vi "FullAlign.vi"(0 "Joystick 0":dbl, 1 "Button":bool=TRUE, 5 "Joystick 1":dbl, 7 "Distance":dbl=-10000.0, 9 "Angle":dbl=-292.57472985881094) -> (4 "Right Motor":dbl=-0.2, 6 "Left Motor":dbl=0.2, 10 "Not In Sight?":bool=TRUE, 15 "In Range?":bool)   [LabVIEW 2016]
uses:
  Systems/Global 1.vi
panel:
  in  "Forward Speed":dbl=0.3 format="%#_13g"
  in  "Max Error":dbl=100.0 format="%#_13g"
  in  "Turn_Gain":dbl=0.25 format="%#_13g"
  in  "Align Effort Addition":dbl=0.175 min=0.0 max=1.0 step=0.05 format="%#_13g"
  in  "Align Target":dbl format="%#_13g"
  in  "MinDistance":dbl=24.0 format="%#_13g"
  out "Sees Target?":bool
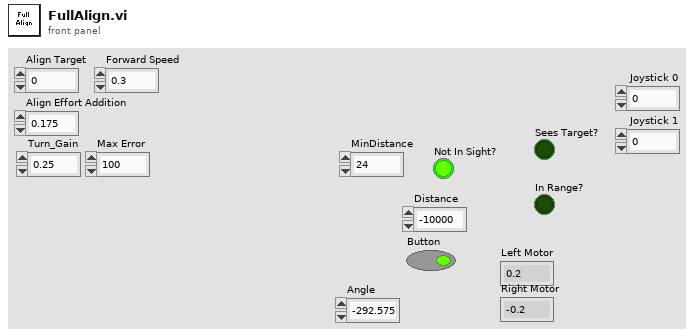
[diagram p1: front panel]
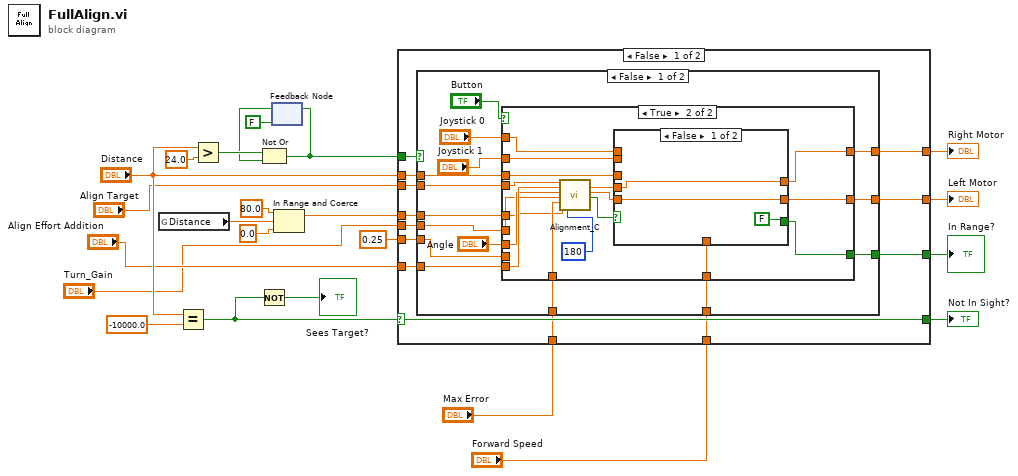
[diagram p0: block diagram]
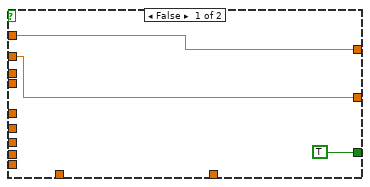
[diagram p2: hidden frame]
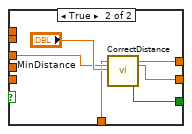
[diagram p3: hidden frame]
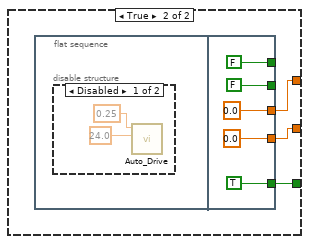
[diagram p4: hidden frame]
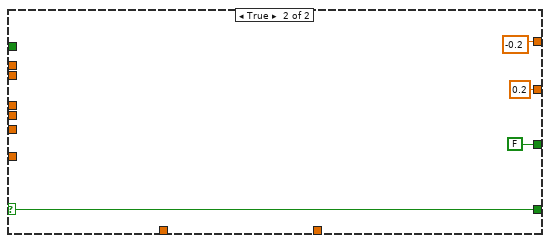
[diagram p6: hidden frame]
diagram:
  n1 = global read "Global 1.vi" "Distance"() -> (w10:dbl)
  n2 = Equal?(x="Distance", y=-10000.0) -> (x = y?=w11:bool)
  n3 = Greater?(x="Distance", y=24.0) -> (0:w16:bool)
  n4 = Not(x=w11) -> (.not. x?=→"Sees Target?":bool)
  n5 = feedback #1(FALSE) -> (w15:bool)
  n6 = Not Or(1:w15, 2:w16) -> (0:w17:bool)
  n7 = feedback-in #1(w17) -> ()
  n8 = In Range and Coerce(upper limit=80.0, x=w10, lower limit=0.0) -> (coerced(x)=w7:dbl)  [unwired: 1 out]
  n9 = case shown="False" w11 {
    selector: w11 -> [w29 w92]
    tunnel: w17 -> [w36 _]
    tunnel: [w35 -0.2] -> w22
    tunnel: [w34 0.2] -> w12
    tunnel: [w33 FALSE] -> w18
    tunnel: "Distance" -> [w32 _]
    tunnel: 0.25 -> [w31 _]
    tunnel: w7 -> [w30 _]
    tunnel: [w29 w92] -> w6
    tunnel: "Align Target" -> [w28 _]
    tunnel: "Align Effort Addition" -> [w27 _]
    tunnel: "Turn_Gain" -> [w26 _]
    tunnel: "Max Error" -> [w25 _]
    tunnel: "Forward Speed" -> [w24 _]
    frame False {
      n10 = case shown="False" w36 {
        tunnel: w32 -> [w47 _]
        tunnel: [w46 w82] -> w35
        tunnel: [w45 w81] -> w34
        tunnel: [w44 w83] -> w33
        tunnel: w31 -> [w43 _]
        tunnel: w30 -> [w42 _]
        tunnel: w28 -> [w41 _]
        tunnel: w27 -> [w40 _]
        tunnel: w26 -> [w39 _]
        tunnel: w25 -> [w38 _]
        tunnel: w24 -> [w37 _]
        frame False {
          n11 = case shown="True" "Button" {
            tunnel: "Joystick 1" -> [w53 w59]
            tunnel: "Joystick 0" -> [w54 w58]
            tunnel: [w53 w71] -> w45
            tunnel: [w54 w70] -> w46
            tunnel: "Angle" -> [_ w65]
            tunnel: [TRUE w69] -> w44
            tunnel: w47 -> [_ w68]
            tunnel: w43 -> [_ _]
            tunnel: w42 -> [_ w61]
            tunnel: w41 -> [_ w67]
            tunnel: w40 -> [_ w66]
            tunnel: w39 -> [_ w64]
            tunnel: w38 -> [_ w63]
            tunnel: w37 -> [_ w57]
            frame False {
            }
            frame True {
              n12 = call "Alignment_C.vi"("Target"=w67, "Effort Addition"=w66, "Camera Feedback"=w65, "Turn_Gain"=w64, "Max Error"=w63, "Range"=w61, "POV"=180) -> ("Right Motor"=w56:dbl, "Left Motor"=w55:dbl, "LeftAndRight?"=w60:bool)  [unwired: 10 in]
              n13 = case shown="False" w60 {
                tunnel: [w72 w79] -> w71
                tunnel: [w73 w78] -> w70
                tunnel: [FALSE w76] -> w69
                tunnel: w68 -> [_ w77]
                tunnel: w59 -> [_ _]
                tunnel: w58 -> [_ _]
                tunnel: w57 -> [_ w75]
                tunnel: w56 -> [w73 _]
                tunnel: w55 -> [w72 _]
                frame False {
                }
                frame True {
                  n14 = call "CorrectDistance.vi"("Speed"=w75, "CenterPoint"="MinDistance", "Distance"=w77) -> ("In Range?"=w76:bool, "Right Motor"=w78:dbl, "Left Motor"=w79:dbl)  [unwired: 22 in]
                }
              }
            }
          }
        }
        frame True {
          n15 = flat-sequence {
            tunnel: [FALSE] -> _
            tunnel: [FALSE] -> _
            tunnel: [TRUE] -> w83
            tunnel: [0.0] -> w82
            tunnel: [0.0] -> w81
            frame #0 {
              n16 = disable-structure shown="Disabled" {
                frame Disabled {
                  n17 = call "Auto_Drive.vi"("distance"=24.0, "Drive Effort"=0.25) -> ()  [unwired: 10 in]
                }
                frame Enabled {
                }
              }
            }
            frame #1 {
            }
          }
        }
      }
    }
    frame True {
    }
  }
  "Right Motor" <- w22
  "Left Motor" <- w12
  "In Range?" <- w18
  "Not In Sight?" <- w6
